vi "Get Target Info.vi"(8 "error in (no error)":errorcluster, 11 "Device Reference in":T1=18446744073709551615 format="%.0x") -> (0 "error out":errorcluster, 2 "Target Info":T2, 3 "Device Reference out":T1=18446744073709551615 format="%.0x")   [LabVIEW 2019, in "Telemetry Engine.lvlib"]
doc: "This VI reads the Target info like: Number of CPU cores, Total Physical Memory, Target Rate (Hz)."
uses:
  Telemetry Engine.lvlib
  <vilib>/NI VeriStand/Custom Device API/Custom Device Item Ref.ctl
  Types/Target Info.ctl
  <vilib>/nisyscfg/Close (System).vi
  <vilib>/NI_Real-Time Target Support.lvlib
  <resource>/objmgr/nisysapi.rc
  <vilib>/nisyscfg/nisyscfg.lvlib
  <vilib>/NI VeriStand/Custom Device API/Custom Device API.lvlib
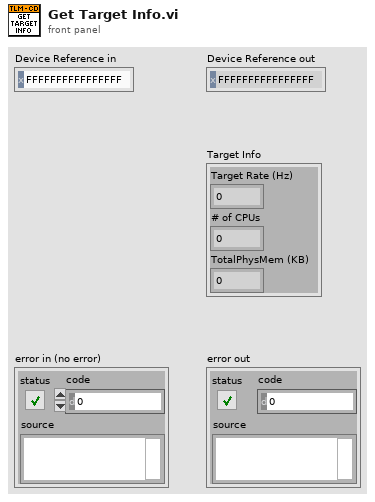
[diagram p1: front panel]
types:
  T1 = typedef "Custom Device API.lvlib/Custom Device Item Ref.ctl" = u64
  T2 = typedef "Telemetry Engine.lvlib/Target Info.ctl" = cluster{"Target Rate (Hz)":dbl, "# of CPUs":u32, "TotalPhysMem (KB)":dbl}
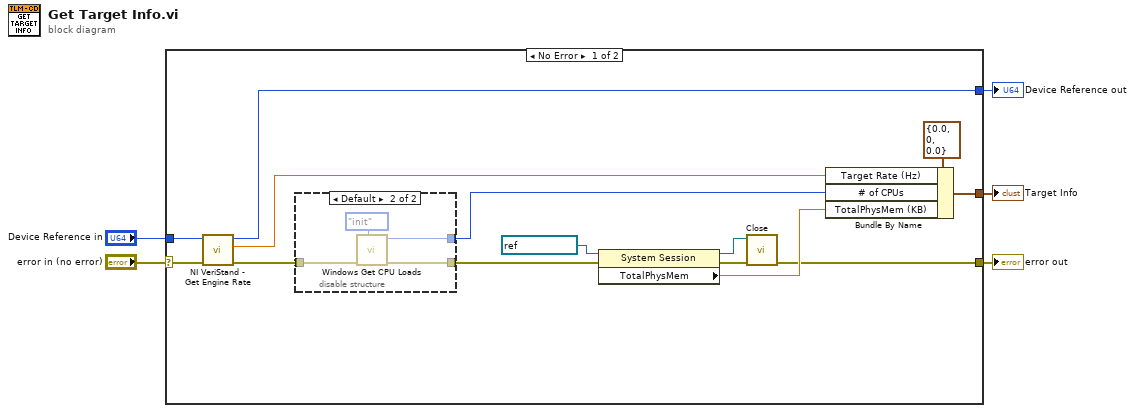
[diagram p0: block diagram]
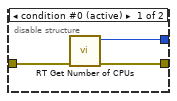
[diagram p2: hidden frame]
diagram:
  n1 = case shown="No Error" "error in (no error)" {
    selector: "error in (no error)" -> [w11 w28]
    tunnel: [w13 _] -> w4
    tunnel: [w12 w28] -> w3
    tunnel: "Device Reference in" -> [w10 w27]
    tunnel: [w9 w27] -> w1
    frame No Error {
      n2 = call <vilib>:"NI VeriStand - Get Engine Rate.vi"("error in (no error)"=w11, "Item Ref in"=w10) -> ("error out"=w7:errorcluster, "Rate (Hz)"=w8:dbl, "Item Ref out"=w9:T1)  [unwired: 7 in]
      n3 = disable-structure shown="Default" {
        disable-tunnel: [w22 w23] -> w15
        disable-tunnel: w7 -> [w21 w26]
        disable-tunnel: [w20 w25] -> w6
        frame condition #0 (active) {
          n4 = call <vilib>:"RT Get Number of CPUs.vi"("error in (no error)"=w21) -> ("error out"=w20:errorcluster, "# of CPUs"=w22:u32)  [unwired: 9 in]
        }
        frame condition #1 {
          n5 = call "Windows Get CPU Loads.vi"("Action"=enum16{"init", "read", "cleanup"}."init", "error in (no error)"=w26) -> ("error out"=w25:errorcluster, "# of CPUs"=w23:u32)  [unwired: 7 in, 1 out]
        }
      }
      n6 = property class="System Session"(reference=refnum<k21> "localhost" ("System Session"), error in=w6) -> (reference out=w18:refnum<k21>, error out=w19:errorcluster, "TotalPhysMem"=w14:dbl)
      n7 = call-poly <vilib>:"Close.vi"("error in (no error)"=w19, "Session in"=w18) -> ("error out"=w12:errorcluster)  [unwired: 9 in]
      n8 = Bundle By Name(cluster=T2 {"Target Rate (Hz)"=0.0, "# of CPUs"=0, "TotalPhysMem (KB)"=0.0} ("Target Info"), "Target Rate (Hz)"=w8, "# of CPUs"=w15, "TotalPhysMem (KB)"=w14) -> (w13:T2)
    }
    frame Error {
    }
  }
  "Target Info" <- w4
  "error out" <- w3
  "Device Reference out" <- w1
